vi "MessageBase.setFieldValue.vi"(8 "error in (no error)":errorcluster, 9 "Value":T1, 10 "FIeld.Name":string="Length", 11 "MessageBase in":refnum<class "MessageBase.lvclass">) -> (0 "error out":errorcluster, 3 "MessageBase out":refnum<class "MessageBase.lvclass">)   [LabVIEW 2022 SP3, in "MessageBase.lvclass"]
uses:
  MessageBase.lvclass
  FieldValue.ctl
  MessageBase.lvclass/MessageBase.ctl
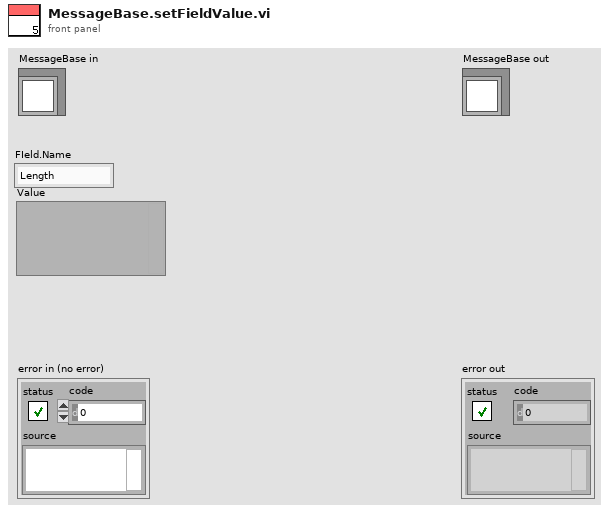
[diagram p1: front panel]
types:
  T1 = typedef "FieldValue.ctl" = variant
  T2 = typedef "FieldSpec.ctl" = cluster{"Name":string, "Offset":i32, "Length":i32, "FieldType":enum16{"Alphanumeric", "Binary", "BinaryLongPrice", "BinaryShortPrice", "BitField", "PrintableAscii", "Value"}, "FieldValue":variant}
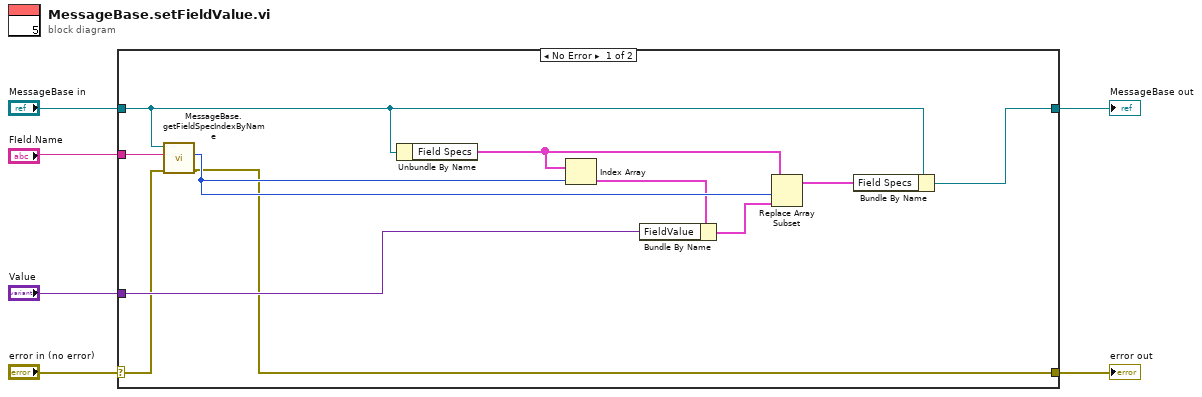
[diagram p0: block diagram]
diagram:
  n1 = case shown="No Error" "error in (no error)" {
    selector: "error in (no error)" -> [w8 w18]
    tunnel: [w7 w18] -> w5
    tunnel: [w9 w19] -> w3
    tunnel: "MessageBase in" -> [w10 w19]
    tunnel: "FIeld.Name" -> [w16 _]
    tunnel: "Value" -> [w12 _]
    frame No Error {
      n2 = call-dynamic "MessageBase.getFieldSpecIndexByName.vi"("error in (no error)"=w8, "Field.Name"=w16, "MessageBase in"=w10) -> ("error out"=w7:errorcluster, "Index"=w14:i32)  [unwired: 6 in, 1 out]
      n3 = Unbundle By Name(w10) -> ("Field Specs"=w15:T2[])
      n4 = Index Array(array=w15, index=w14) -> (element=w13:T2)
      n5 = Bundle By Name(cluster=w13, "FieldValue"=w12) -> (w11:T2)
      n6 = Replace Array Subset(array=w15, new element=w11, index=w14) -> (w17:T2[])
      n7 = Bundle By Name(cluster=w10, "Field Specs"=w17) -> (w9:refnum<class "MessageBase.lvclass">)
    }
    frame Error {
      # "Wire the error cluster across even in the \"No Error\"\ncase so that warnings get propagated."
    }
  }
  "error out" <- w5
  "MessageBase out" <- w3
